vi "DSF.Engine.Transfer.Get String Buffer.vi"(11 "Transfer in":refnum<class "DSF.Engine.Transfer.lvclass">) -> (2 "Buffer":refnum<class "DSF.Engine.Memory.Buffer.lvclass">, 3 "Transfer out":refnum<class "DSF.Engine.Transfer.lvclass">)   [LabVIEW 2017, in "Data Sharing Framework Engine.lvlib" / "DSF.Engine.Transfer.lvclass"]
uses:
  DSF.Engine.Transfer.lvclass
  Buffer/DSF.Engine.Memory.Buffer.lvclass
  DSF.Engine.Transfer.lvclass/DSF.Engine.Transfer.ctl
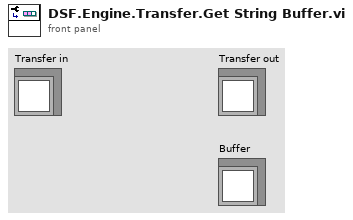
[diagram p1: front panel]
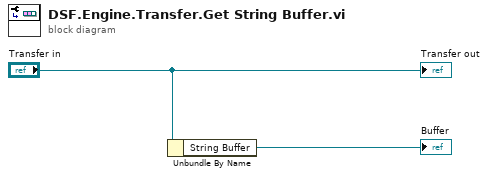
[diagram p0: block diagram]
diagram:
  n1 = Unbundle By Name("Transfer in") -> ("String Buffer"=→"Buffer":refnum<class "DSF.Engine.Memory.Buffer.lvclass">)
  "Transfer out" <- "Transfer in"
